vi "Set Home State.vi"(8 "error in (no error)":errorcluster, 9 "Home?":bool, 10 "Motor":i32, 11 "Filter Wheel in":refnum<class "Filter Wheel.lvclass">) -> (0 "error out":errorcluster, 3 "Filter Wheel out":refnum<class "Filter Wheel.lvclass">)   [LabVIEW 2024, in "Filter Wheel.lvclass"]
uses:
  Filter Wheel.lvclass
  Filter Wheel.lvclass/Filter Wheel.ctl
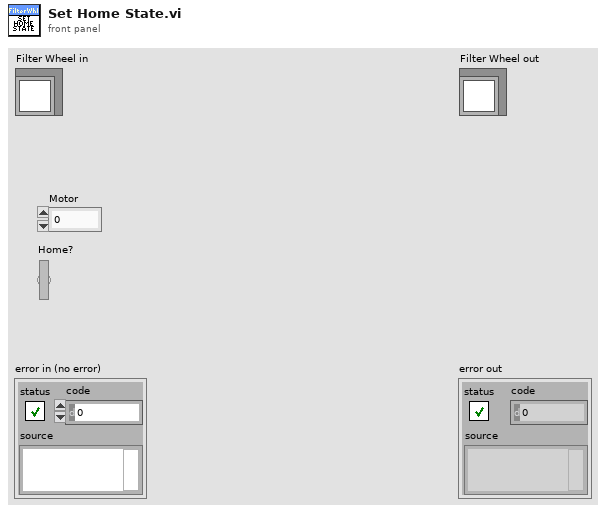
[diagram p1: front panel]
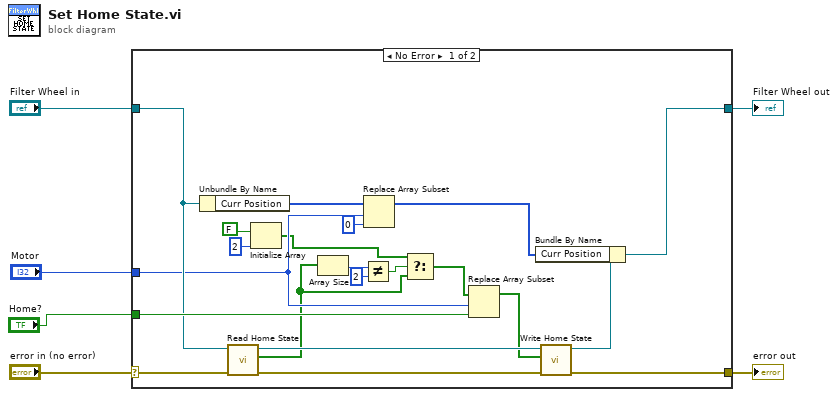
[diagram p0: block diagram]
diagram:
  n1 = case shown="No Error" "error in (no error)" {
    selector: "error in (no error)" -> [w25 w29]
    tunnel: [w23 w29] -> w5
    tunnel: [w20 w28] -> w3
    tunnel: "Filter Wheel in" -> [w19 w28]
    tunnel: "Motor" -> [w17 _]
    tunnel: "Home?" -> [w22 _]
    frame No Error {
      n2 = Unbundle By Name(w19) -> ("Curr Position"=w18:i32[])
      n3 = call-dynamic "Read Home State.vi"("error in (no error)"=w25, "Filter Wheel in"=w19) -> ("error out"=w24:errorcluster, "Home State"=w11:bool[], "Filter Wheel out"=w27:refnum<class "Filter Wheel.lvclass">)  [unwired: 7 in]
      n4 = Initialize Array(FALSE, 2 ("dimension size")) -> (w7:bool[])
      n5 = Array Size(array=w11) -> (size(s)=w14:i32)
      n6 = Not Equal?(x=w14, y=2) -> (x != y?=w12:bool)
      n7 = Replace Array Subset(array=w18, new element=0 ("new element/subarray"), index=w17) -> (w15:i32[])
      n8 = Select(t=w7, s=w12, f=w11) -> (s? t:f=w10:bool[])
      n9 = Replace Array Subset(array=w10, new element=w22, index=w17) -> (w26:bool[])
      n10 = call-dynamic "Write Home State.vi"("error in (no error)"=w24, "Home State"=w26, "Filter Wheel in"=w27) -> ("error out"=w23:errorcluster, "Filter Wheel out"=w21:refnum<class "Filter Wheel.lvclass">)  [unwired: 7 in]
      n11 = Bundle By Name(cluster=w21, "Curr Position"=w15) -> (w20:refnum<class "Filter Wheel.lvclass">)
    }
    frame Error {
    }
  }
  "error out" <- w5
  "Filter Wheel out" <- w3
